vi "Get Owner of Type.vi"(7 "Match Type":enum16{"Exact Match", "Contains"}(ring), 8 "error in":errorcluster, 10 "Owner Class Name desired":string, 11 "reference":refnum<vi>) -> (0 "error out":errorcluster, 1 "Owner heirarchy":string[](array[string]), 2 "Owner of type found?":bool, 3 "Owner of Type":refnum<vi>, 4 "ClassName of ref returned":string)   [LabVIEW 2023]
doc: "Input is a generic Reference (any Gobject) and the output is the class heirarchy, as well as the first owner ref to match a given input value.\n\nExact match is entire class name (case insensitive).\n\nContains Match would return the TopLevelDiagram class if \"Diagram\" were input (case insensitive), unless the input object is in a subdiagram, such as inside a sequence structure, in which case that diagram ref would be returned."
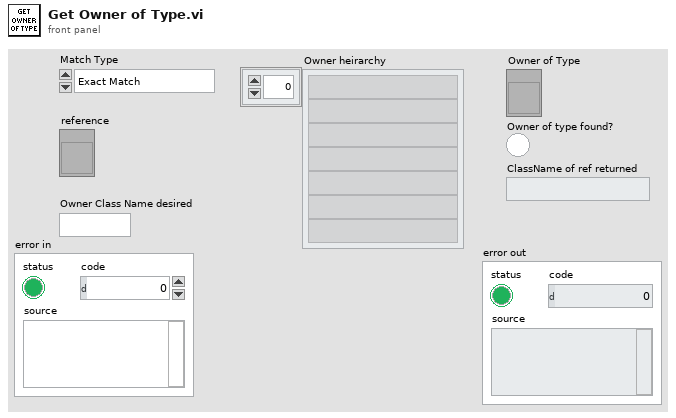
[diagram p1: front panel]
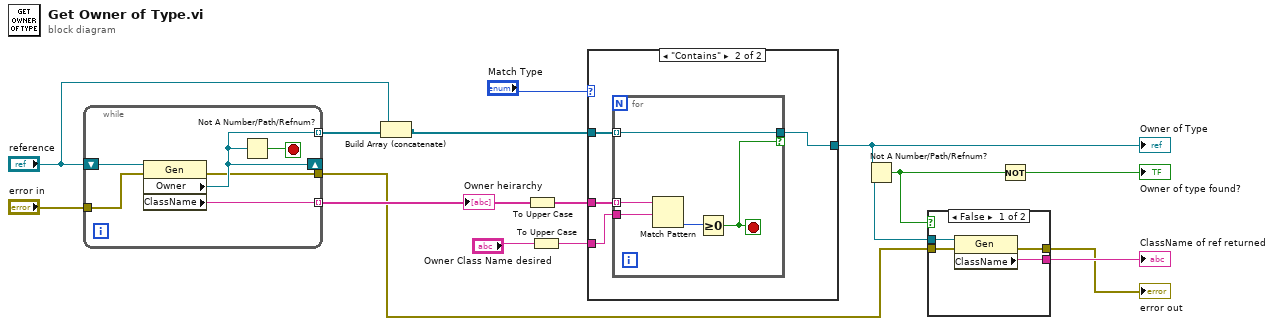
[diagram p0: block diagram]
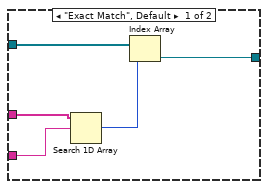
[diagram p3: hidden frame]
diagram:
  n1 = while {
    shift-right: [w18] -> _
    shift-left: "reference" -> [w21]
    tunnel: [w20] -> w4 mode=indexing
    tunnel: [w18] -> w8 mode=indexing
    tunnel: "error in" -> [w17]
    tunnel: [w16] -> w2
    stop <- w19 stop-if-true
    n2 = property class="Gen"(reference=w21, error in=w17) -> (error out=w16:errorcluster, "Owner"=w18:refnum<vi>, "ClassName"=w20:string)  [unwired: 1 out]
    n3 = Not A Number/Path/Refnum?(number/path/refnum=w18) -> (NaN/Path/Refnum?=w19:bool)
  }
  "Owner heirarchy" <- w4
  n4 = Build Array (concatenate)("reference", w8) -> (w6:refnum<vi>[])
  n5 = To Upper Case(1:w4) -> (0:w13:string[])
  n6 = To Upper Case(1:"Owner Class Name desired") -> (0:w12:string)
  n7 = case shown="\"Contains\"" "Match Type" {
    tunnel: w13 -> [w23 w30]
    tunnel: w12 -> [w26 w29]
    tunnel: w6 -> [w25 w28]
    tunnel: [w24 w27] -> w10
    frame "Exact Match", Default {
      n8 = Search 1D Array(1D array=w23, element=w26) -> (index of element=w22:i32)  [unwired: 1 in]
      n9 = Index Array(array=w25, index=w22) -> (element=w24:refnum<vi>)
    }
    frame "Contains" {
      n10 = for {
        tunnel: w30 -> [w35] mode=indexing
        tunnel: w29 -> [w34]
        tunnel: [w32] -> w27 if=w31
        tunnel: w28 -> [w32] mode=indexing
        stop <- w31 stop-if-true
        n11 = Match Pattern(string=w35, regular expression=w34) -> (offset past match=w33:i32)  [unwired: 1 in, 3 out]
        n12 = Greater Or Equal To 0?(x=w33) -> (x >= 0?=w31:bool)
      }
    }
  }
  "Owner of Type" <- w10
  n13 = Not A Number/Path/Refnum?(number/path/refnum=w10) -> (NaN/Path/Refnum?=w5:bool)
  n14 = case shown="False" w5 {
    tunnel: w10 -> [w39 _]
    tunnel: [w38 _] -> w9
    tunnel: w2 -> [w37 w40]
    tunnel: [w36 w40] -> w1
    frame False {
      n15 = property class="Gen"(reference=w39, error in=w37) -> (error out=w36:errorcluster, "ClassName"=w38:string)  [unwired: 1 out]
    }
    frame True {
    }
  }
  "ClassName of ref returned" <- w9
  "error out" <- w1
  n16 = Not(x=w5) -> (.not. x?=→"Owner of type found?":bool)
